vi "IsEnabled.vi"(8 "error in (no error)":errorcluster, 11 "QuickControl in":refnum<class "QuickSilver.lvclass">) -> (0 "error out":errorcluster, 2 "Boolean":bool, 3 "QuickControl out":refnum<class "QuickSilver.lvclass">)   [LabVIEW 2018, in "QuickSilver.lvclass"]
uses:
  QuickSilver.lvclass
  QuickSilver.lvclass/QuickSilver.ctl
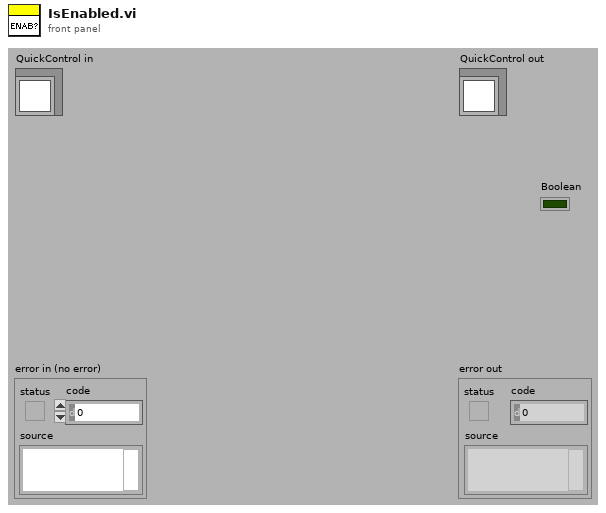
[diagram p1: front panel]
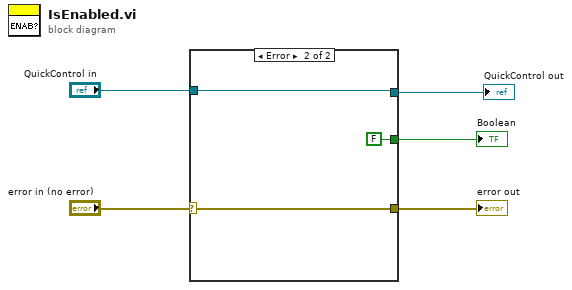
[diagram p0: block diagram]
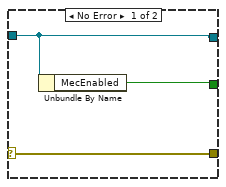
[diagram p2: hidden frame]
diagram:
  n1 = case shown="Error" "error in (no error)" {
    selector: "error in (no error)" -> [w6 w9]
    tunnel: "QuickControl in" -> [w8 w10]
    tunnel: [w6 w9] -> w3
    tunnel: [w8 w10] -> w2
    tunnel: [w7 FALSE ("MecEnabled")] -> w1
    frame No Error {
      n2 = Unbundle By Name(w8) -> ("MecEnabled"=w7:bool)
    }
    frame Error {
    }
  }
  "error out" <- w3
  "QuickControl out" <- w2
  "Boolean" <- w1
